vi "AIT 664 - Separate Tx-Rx Messages.vi"(8 "error in (no error)":errorcluster, 11 "HW Channel - Section in":T1 {"Message Settings"."Driver Data"."First Word" min=8 max=31; "Message Settings"."Driver Data"."Num Bits" min=1 max=32; "Message Settings"."Driver Data"."Start Bit" min=8 max=31; "Message Settings"."Block Data Refs"."Data Reference" format="%.0x"; "Rx Com Udp Port"."Handle" format="%08x"; "Tx Com Udp Port"."Handle" format="%08x"}) -> (0 "error out":errorcluster, 2 "HW Channel Rx - Section out":T1 {"Message Settings"."Driver Data"."First Word" min=8 max=31; "Message Settings"."Driver Data"."Num Bits" min=1 max=32; "Message Settings"."Driver Data"."Start Bit" min=8 max=31; "Message Settings"."Block Data Refs"."Data Reference" format="%.0x"; "Rx Com Udp Port"."Handle" format="%08x"; "Tx Com Udp Port"."Handle" format="%08x"}, 3 "HW Channel Tx - Section out":T1 {"Message Settings"."Driver Data"."First Word" min=8 max=31; "Message Settings"."Driver Data"."Num Bits" min=1 max=32; "Message Settings"."Driver Data"."Start Bit" min=8 max=31; "Message Settings"."Block Data Refs"."Data Reference" format="%.0x"; "Rx Com Udp Port"."Handle" format="%08x"; "Tx Com Udp Port"."Handle" format="%08x"})   [LabVIEW 2013, in "AIT 664 Custom Device.lvlib"]
uses:
  AIT 664 Custom Device.lvlib
  Controls and Global/Number of Bits.ctl
  Controls and Global/Start Bit.ctl
  RT Controls/AIT 664 - Driver Data.ctl
  <vilib>/NI Veristand/Custom Device API/Data Reference.ctl
  <vilib>/NI Veristand/Custom Device API/Custom Device API.lvlib
  <vilib>/NI Veristand/Custom Device API/Block Data Reference.ctl
  RT Controls/AIT 664 - RT Message Settings.ctl
  RT Controls/AIT 664 - RT Hardware Channel.ctl
  <userlib>/ARINC 664/AIT 664 Controls/General/Direction.ctl
  <userlib>/ARINC 664/AIT 664 API.lvlib
  <userlib>/ARINC 664/AIT 664 Controls/General/Message Port Type.ctl
  <userlib>/ARINC 664/AIT 664 Controls/General/Message Port.ctl
  System Explorer/Controls/664 - Sampling Type.ctl
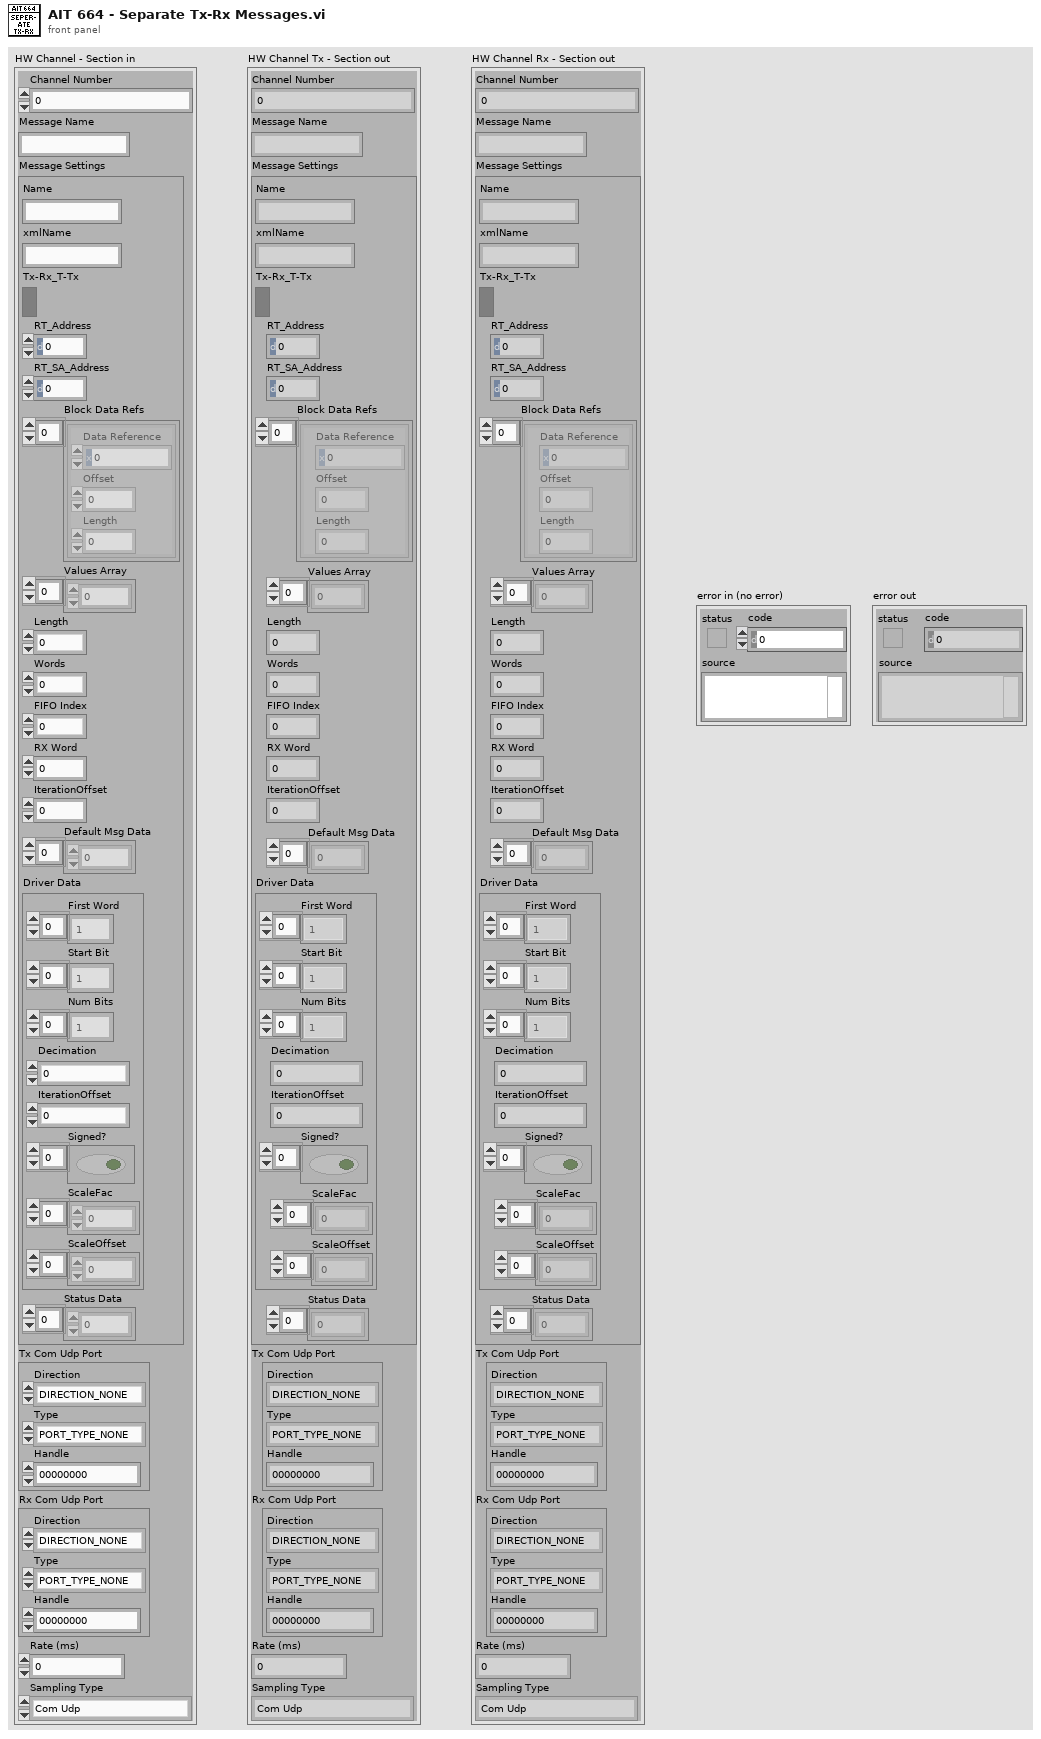
[diagram p1: front panel]
types:
  T1 = typedef "AIT 664 Custom Device.lvlib/AIT 664 - RT Hardware Channel.ctl" = cluster{"Channel Number":u16, "Message Name":string, "Message Settings":T2, "Tx Com Udp Port":T8, "Rx Com Udp Port":T8, "Rate (ms)":u32, "Sampling Type":T11}
  T2 = typedef "AIT 664 Custom Device.lvlib/AIT 664 - RT Message Settings.ctl" = cluster{"Name":string, "xmlName":string, "Tx-Rx_T-Tx":bool, "RT_Address":u8, "RT_SA_Address":u8, "Block Data Refs":T3[], "Values Array":dbl[], "Length":i32, "Words":i32, "FIFO Index":i32, "RX Word":u32, "IterationOffset":i32, "Default Msg Data":u8[], "Driver Data":T5, "Status Data":u32[]}
  T3 = typedef "Custom Device API.lvlib/Block Data Reference.ctl" = cluster{"Data Reference":T4, "Offset":i32, "Length":i32}
  T4 = typedef "Custom Device API.lvlib/Data Reference.ctl" = i32
  T5 = typedef "AIT 664 Custom Device.lvlib/AIT 664 - Driver Data.ctl" = cluster{"First Word":T6[], "Start Bit":T6[], "Num Bits":T7[], "Decimation":i32, "IterationOffset":i32, "Signed?":bool[], "ScaleFac":dbl[], "ScaleOffset":dbl[]}
  T6 = typedef "AIT 664 Custom Device.lvlib/Start Bit.ctl" = i32
  T7 = typedef "AIT 664 Custom Device.lvlib/Number of Bits.ctl" = i32
  T8 = typedef "AIT 664 API.lvlib/Message Port.ctl" = cluster{"Direction":T9, "Type":T10, "Handle":u64}
  T9 = typedef "AIT 664 API.lvlib/Direction.ctl" = enum16{"DIRECTION_NONE", "DIRECTION_TX", "DIRECTION_RX"}
  T10 = typedef "AIT 664 API.lvlib/Message Port Type.ctl" = enum16{"PORT_TYPE_NONE", "COM_UDP", "SAP_UDP", "SAP_IP", "SAP_MAC", "COTS_MAC", "COTS_MAC_RAW"}
  T11 = typedef "AIT 664 Custom Device.lvlib/664 - Sampling Type.ctl" = enum16{"Com Udp", "Com Udp Queuing", "Sap Udp", "Sap Ip", "Sap Mac", "Unknown"}
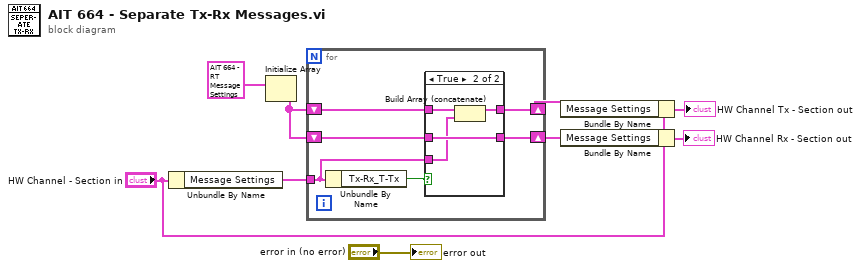
[diagram p0: block diagram]
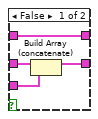
[diagram p2: hidden frame]
diagram:
  n1 = Unbundle By Name("HW Channel - Section in") -> ("Message Settings"=w3:T2)
  n2 = Initialize Array(T2 {"Name"="", "xmlName"="", "Tx-Rx_T-Tx"=FALSE, "RT_Address"=0, "RT_SA_Address"=0, "Block Data Refs"=[], "Values Array"=[], "Length"=0, "Words"=0, "FIFO Index"=0, "RX Word"=0, "IterationOffset"=0, "Default Msg Data"=[], "Driver Data"={"First Word"=[], "Start Bit"=[], "Num Bits"=[], "Decimation"=0, "IterationOffset"=0, "Signed?"=[], "ScaleFac"=[], "ScaleOffset"=[]}, "Status Data"=[]} ("Message Settings")) -> (w5:T2[])  [unwired: 1 in]
  n3 = for {
    shift-right: [w10] -> w8
    shift-left: w5 -> [w13]
    shift-right: [w11] -> w7
    shift-left: w5 -> [w12]
    tunnel: w3 -> [w14]
    n4 = Unbundle By Name(w14) -> ("Tx-Rx_T-Tx"=w15:bool)
    n5 = case shown="True" w15 {
      tunnel: w14 -> [w18 w21]
      tunnel: w13 -> [w17 w22]
      tunnel: w12 -> [w19 w23]
      tunnel: [w16 w23] -> w11
      tunnel: [w17 w20] -> w10
      frame False {
        n6 = Build Array (concatenate)(w19, w18) -> (w16:T2[])
      }
      frame True {
        n7 = Build Array (concatenate)(w22, w21) -> (w20:T2[])
      }
    }
  }
  n8 = Bundle By Name(cluster="HW Channel - Section in", "Message Settings"=w8) -> (→"HW Channel Tx - Section out":T1)
  n9 = Bundle By Name(cluster="HW Channel - Section in", "Message Settings"=w7) -> (→"HW Channel Rx - Section out":T1)
  "error out" <- "error in (no error)"
